vi "ADQ214 Write Register.vi"(6 "data":i32, 7 "mask":i32, 8 "error in (no error)":errorcluster, 9 "addr":i32, 10 "ADQ214_num":i32, 11 "adq_cu_ptr":u32) -> (0 "error out":errorcluster, 2 "function return":u32, 3 "adq_cu_ptr out":u32)   [LabVIEW 8.6, in "ADQAPI.lvlib"]
doc: "extern \"C\" __declspec(dllimport) unsigned int ADQ214_WriteRegister(void* adq_cu_ptr, int ADQ214_num, int addr, int mask, int data);"
uses:
  F/HRT/Sp Devices Thesis/ADQ-214 project (H R)/ADQAPI.lvlib
  F:/HRT/Sp Devices Thesis/ADQ-214 project (H R)/ADQAPI.dll
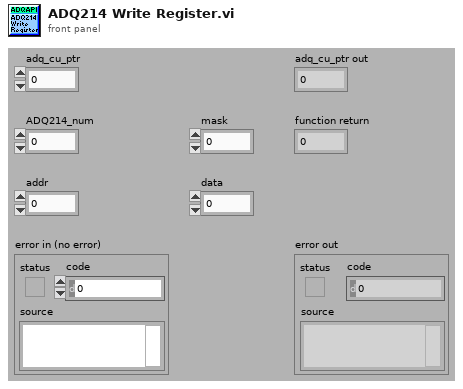
[diagram p1: front panel]
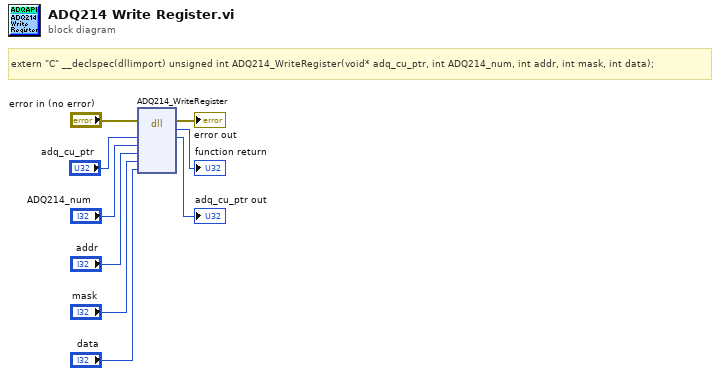
[diagram p0: block diagram]
diagram:
  # "extern \"C\" __declspec(dllimport) unsigned int\tADQ214_WriteRegister(void* adq_cu_ptr, int ADQ214_num, int addr, int mask, int data);"
  n1 = dll-call lib="F:/HRT/Sp Devices Thesis/ADQ-214 project (H R)/ADQAPI.*" fn="ADQ214_WriteRegister"(error in="error in (no error)", "adq_cu_ptr"="adq_cu_ptr", "ADQ214_num"="ADQ214_num", "addr"="addr", "mask"="mask", "data"="data") -> (error out=→"error out":errorcluster, →"function return":u32, "adq_cu_ptr"=→"adq_cu_ptr out":u32)  [unwired: 6 in, 1 out]
